vi "Get Array Cycle (subVI).vi"(10 "Marker":dbl=inf, 11 "Array Samples":dbl[](array[numeric])) -> (2 "Found?":bool, 3 "Array":dbl[](array[numeric]))   [LabVIEW 2020]
uses:
  <userlib>/_OpenG.lib/array/array.llb/Search 1D Array (DBL)__ogtk.vi
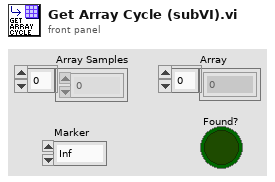
[diagram p1: front panel]
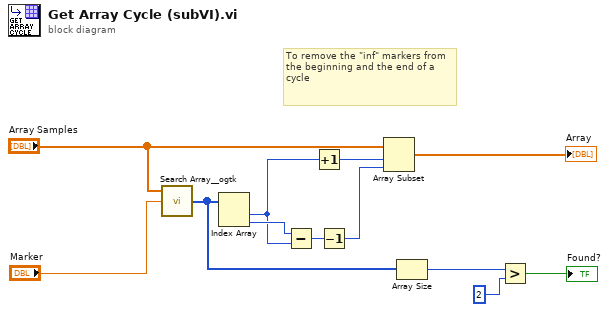
[diagram p0: block diagram]
diagram:
  # "To remove the \"inf\" markers from the beginning and the end of a cycle"
  n1 = call-poly <userlib>:"Search Array__ogtk.vi"("Array"="Array Samples", "Element Data"="Marker") -> ("Indices of Elements"=w6:i32[])  [unwired: 7 in]
  n2 = Index Array(array=w6) -> (element #1=w2:i32, element #2=w8:i32)  [unwired: 2 in]
  n3 = Subtract(x=w8, y=w2) -> (x-y=w10:i32)
  n4 = Increment(x=w2) -> (x+1=w1:i32)
  n5 = Decrement(x=w10) -> (x-1=w11:i32)
  n6 = Array Subset(array="Array Samples", index=w1, length=w11) -> (→"Array":dbl[])
  n7 = Array Size(array=w6) -> (size(s)=w5:i32)
  n8 = Greater?(x=w5, y=2) -> (0:→"Found?":bool)
